vi "GenNet Close Connection.vi"(8 "error in (no error)":errorcluster, 11 "TCP Network Connection in":refnum<k5>) -> (0 "error out":errorcluster, 3 "TCP Network Connection out":refnum<k5>)   [LabVIEW 2020, in "hse-gennet.lvlib"]
doc: "Closes a TCP/IP connection.\n\n____\nHAMPEL SOFTWARE ENGINEERING v3.8.0 (2023-12-18 14:41)"
uses:
  hse-gennet.lvlib
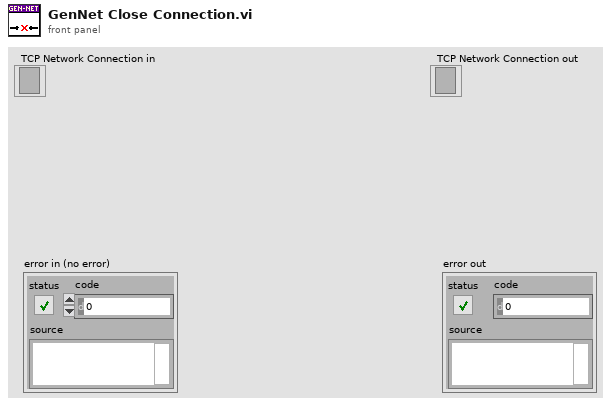
[diagram p1: front panel]
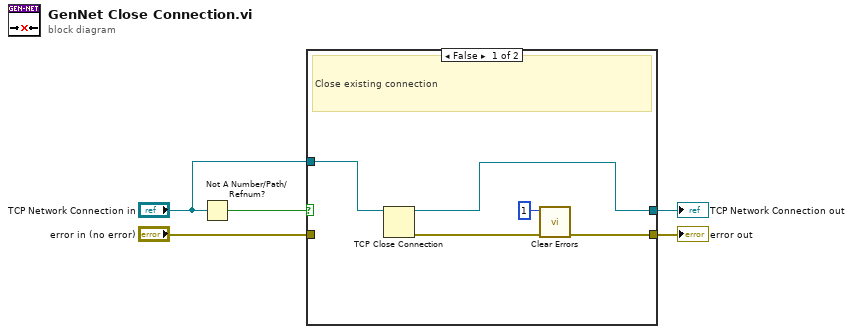
[diagram p0: block diagram]
diagram:
  n1 = Not A Number/Path/Refnum?(number/path/refnum="TCP Network Connection in") -> (NaN/Path/Refnum?=w1:bool)
  n2 = case shown="False" w1 {
    tunnel: [w6 w11] -> w5
    tunnel: [w9 w12] -> w4
    tunnel: "error in (no error)" -> [_ w12]
    tunnel: "TCP Network Connection in" -> [w7 w11]
    frame False {
      # "Close existing connection"
      n3 = TCP Close Connection(connection ID=w7) -> (connection ID out=w6:refnum<k5>, error out=w10:errorcluster)  [unwired: 1 in, 1 out]
      n4 = call <vilib>:"Clear Errors.vi"("error in (no error)"=w10, "specific error code to clear (0: all)"=1) -> ("error out"=w9:errorcluster)  [unwired: 4 in, 1 out]
    }
    frame True {
      # "invalid connection reference - do nothing"
    }
  }
  "TCP Network Connection out" <- w5
  "error out" <- w4
